vi "AC Output.vi"(0 "Scope In":string, 5 "Channel":i32, 11 "Error In":errorcluster) -> (4 "Waveform Data":dbl[](array[numeric]), 6 "Frequency":dbl, 8 "Amplitude":dbl, 10 "Phase":dbl, 15 "Error Out":errorcluster)   [LabVIEW 2015]
doc: "Measure the frequency of the AC signal. Before calling this VI, ensure that the input signal is set for the battery pin."
uses:
  <vilib>/measure/matone.llb/Extract Single Tone Information 1 Chan.vi
  <instrlib>/Driver Simulation/Oscilloscope.lvlib
  <vilib>/measure/NI_MAPro.lvlib
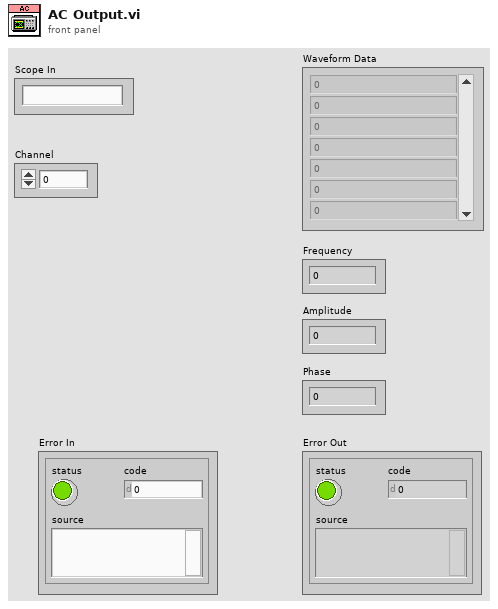
[diagram p1: front panel]
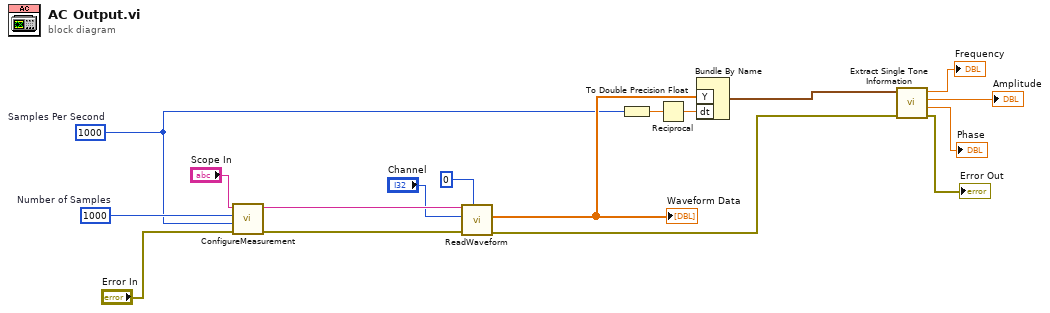
[diagram p0: block diagram]
diagram:
  w3 = 1000  # Samples Per Second
  w7 = 1000  # Number of Samples
  n1 = call <instrlib>:"ConfigureMeasurement.vi"("error in (no error)"="Error In", "Samples Per Second"=w3, "Number of Samples"=w7, "Scope in"="Scope In") -> ("error out"=w16:errorcluster, "Scope out"=w17:string)  [unwired: 6 in]
  n2 = call <instrlib>:"ReadWaveform.vi"("Test Socket (0)"=0, "error in (no error)"=w16, "Channel"="Channel", "Scope in"=w17) -> ("error out"=w8:errorcluster, "Result"=w14:dbl[])  [unwired: 5 in, 1 out]
  "Waveform Data" <- w14
  n3 = To Double Precision Float(number=w3) -> (double precision float=w4:dbl)
  n4 = Reciprocal(x=w4) -> (1/x=w5:dbl)
  n5 = Bundle By Name("Y"=w14, "dt"=w5) -> (w13:waveform(dbl))  [unwired: 1 in]
  n6 = call-poly <vilib>:"Extract Single Tone Information.vi"("error in (no error)"=w8, "time signal in"=w13) -> ("error out"=→"Error Out":errorcluster, "detected phase (deg)"=→"Phase":dbl, "detected amplitude"=→"Amplitude":dbl, "detected frequency"=→"Frequency":dbl)  [unwired: 4 in, 2 out]
